vi "findZerosAndInterpolate.vi"(0 "Waveform":waveform(dbl)) -> (1 "Waveform out spline":waveform(dbl)(graph), 2 "missing indices":i32[][](array[numeric]))   [LabVIEW 2017]
uses:
  <vilib>/gmath/NI_Gmath.lvlib
panel:
  out "Waveform Graph":waveform(dbl)(graph)
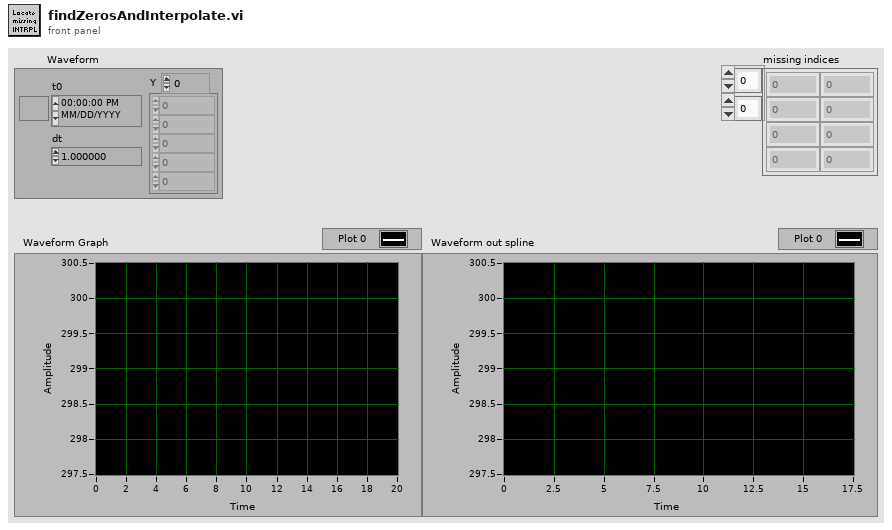
[diagram p1: front panel]
types:
  T1 = cluster{"boundary":enum16{"natural spline", "not-a-knot", "1st derivative", "2nd derivative"}, "derivative value":dbl}
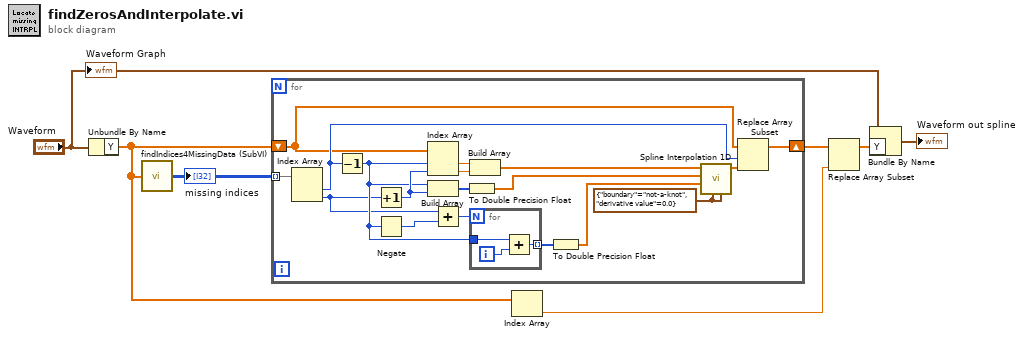
[diagram p0: block diagram]
diagram:
  n1 = Unbundle By Name("Waveform") -> ("Y"=w2:dbl[])
  n2 = call "findIndices4MissingData (SubVI).vi"("data"=w2) -> ("missing data indices"=w7:i32[][])
  "missing indices" <- w7
  n3 = for {
    tunnel: w7 -> [w25] mode=indexing
    shift-right: [w13] -> w5
    shift-left: w2 -> [w11]
    w22 = T1 {"boundary"=enum."not-a-knot", "derivative value"=0.0} ("initial boundary")
    n4 = Index Array(array=w25) -> (element #1=w12:i32, element #2=w9:i32)  [unwired: 2 in]
    n5 = Decrement(x=w12) -> (x-1=w10:i32)
    n6 = Increment(x=w9) -> (x+1=w21:i32)
    n7 = Negate(x=w10) -> (-x=w8:i32)
    n8 = Index Array(array=w11, index #1=w10, index #2=w21) -> (element #1=w24:dbl, element #2=w23:dbl)
    n9 = Build Array(w10, w21) -> (w20:i32[])
    n10 = Add(x=w9, y=w8) -> (x+y=w17:i32)
    n11 = To Double Precision Float(number=w20) -> (double precision float=w18:dbl[])
    n12 = Build Array(w24, w23) -> (w19:dbl[])
    n13 = for {
      N: w17 -> [_]
      tunnel: w10 -> [w28]
      tunnel: [w26] -> w16 mode=indexing
      i -> [w27]
      n14 = Add(x=w28, y=w27) -> (x+y=w26:i32)
    }
    n15 = To Double Precision Float(number=w16) -> (double precision float=w15:dbl[])
    n16 = call <vilib>:"Spline Interpolation 1D.vi"("final boundary"=w22, "initial boundary"=w22, "xi"=w15, "X"=w18, "Y"=w19) -> ("yi"=w14:dbl[])  [unwired: 4 in, 2 out]
    n17 = Replace Array Subset(array=w11, new element=w14, index=w12) -> (w13:dbl[])
  }
  n18 = Index Array(array=w2) -> (element=w1:dbl)  [unwired: 1 in]
  n19 = Replace Array Subset(array=w5, new element=w1) -> (w3:dbl[])  [unwired: 1 in]
  n20 = Bundle By Name(cluster="Waveform", "Y"=w3) -> (→"Waveform out spline":waveform(dbl))
  "Waveform Graph" <- "Waveform"
